vi "Not Found Dialog.vi"(1 "Help":string, 2 "Message":string, 3 "Stop":string, 4 "Continue":string, 5 "type of dialog (OK msg:1)":T1) -> (0 "stop event propagated":bool)   [LabVIEW 2020]
uses:
  DialogTypeEnum.ctl
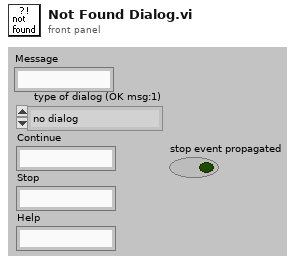
[diagram p1: front panel]
types:
  T1 = typedef "DialogTypeEnum.ctl" = enum16{"no dialog", "OK message", "continue or stop message", "auto error handling dialog", "OK message + warnings", "continue/stop + warnings"}
  T2 = enum16{"Left Button", "Center Button", "Right Button", "Window Close"}
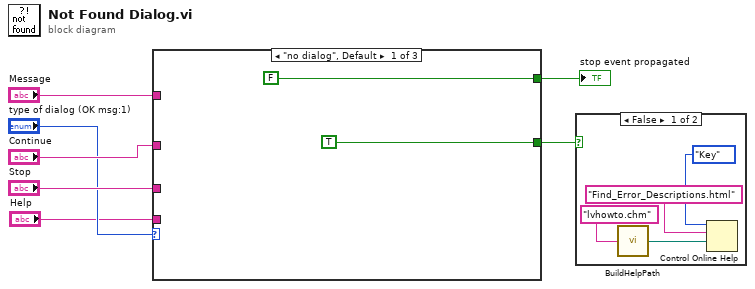
[diagram p0: block diagram]
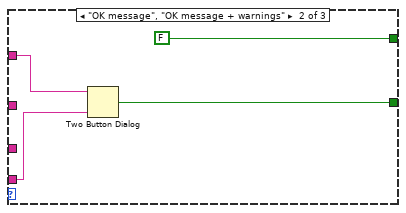
[diagram p3: hidden frame]
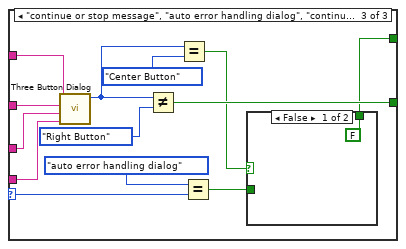
[diagram p4: hidden frame]
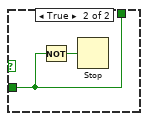
[diagram p5: hidden frame]
diagram:
  n1 = case shown="\"no dialog\", Default" "type of dialog (OK msg:1)" {
    selector: "type of dialog (OK msg:1)" -> [_ _ w17]
    tunnel: "Help" -> [_ w13 w25]
    tunnel: "Message" -> [_ w12 w26]
    tunnel: "Continue" -> [_ _ w24]
    tunnel: "Stop" -> [_ _ w23]
    tunnel: [FALSE FALSE w14] -> w7
    tunnel: [TRUE w10 w22] -> w1
    frame "no dialog", Default {
    }
    frame "OK message", "OK message + warnings" {
      n2 = Two Button Dialog(message=w12, 1:w13) -> (T button?=w10:bool)  [unwired: 1 in]
    }
    frame "continue or stop message", "auto error handling dialog", "continue/stop + warnings" {
      n3 = call "Three Button Dialog.vi"("Right Button Text (\"Cancel\")"=w25, "Center Button Text (\"No\")"=w23, "Left Button Text (\"Yes\")"=w24, "message"=w26) -> ("Which Button?"=w20:T2)  [unwired: 7 in]
      n4 = Not Equal?(x=w20, y=T2."Right Button" ("Which Button?")) -> (x != y?=w22:bool)
      n5 = Equal?(x=w20, y=T2."Center Button" ("Which Button?")) -> (x = y?=w16:bool)
      n6 = Equal?(x=DialogTypeEnum."auto error handling dialog" ("type of dialog (OK msg:1)"), y=w17) -> (x = y?=w15:bool)
      n7 = case shown="False" w16 {
        tunnel: w15 -> [_ w29]
        tunnel: [FALSE w29] -> w14
        frame False {
        }
        frame True {
          n8 = Not(x=w29) -> (.not. x?=w28:bool)
          n9 = Stop(stop? (T)=w28) -> ()
        }
      }
    }
  }
  "stop event propagated" <- w7
  n10 = case shown="False" w1 {
    frame False {
      n11 = call "BuildHelpPath.vi"("Help File Name"="lvhowto.chm") -> ("Help File Path"=w31:path)
      n12 = Control Online Help(2:w31, 3:"Find_Error_Descriptions.html" ("String to search for"), 4:enum16{"Contents", "Key", "Close"}."Key" ("Operation")) -> ()  [unwired: 1 in, 1 out]
    }
    frame True {
    }
  }
